vi "pop camera error.vi"(8 "error in (no error)":errorcluster, 11 "Channel in":refnum<class "Channel.lvclass">) -> (0 "error out":errorcluster, 2 "error":errorcluster, 3 "Channel out":refnum<class "Channel.lvclass">)   [LabVIEW 2018, in "Channel.lvclass"]
uses:
  Channel.lvclass
  Channel.lvclass/Channel.ctl
  Simulated_CCD_Camera/Simulated Camera.lvclass/Simulated Camera.ctl
  Simulated_CCD_Camera/Simulated Camera.lvclass
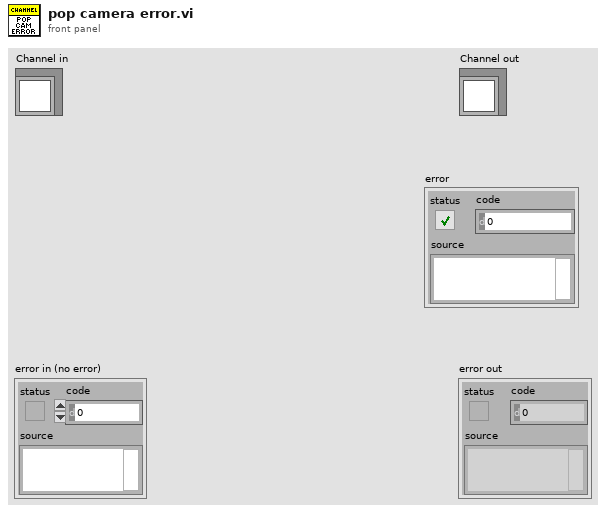
[diagram p1: front panel]
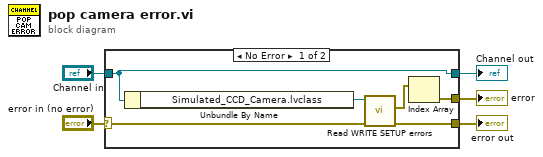
[diagram p0: block diagram]
diagram:
  n1 = case shown="No Error" "error in (no error)" {
    selector: "error in (no error)" -> [w9 w13]
    tunnel: [w8 w13] -> w4
    tunnel: [w11 w12] -> w2
    tunnel: "Channel in" -> [w11 w12]
    tunnel: [w6 _] -> w1
    frame No Error {
      n2 = Unbundle By Name(w11) -> ("Simulated_CCD_Camera.lvclass"=w10:refnum<class "Simulated Camera.lvclass">)
      n3 = call "Read WRITE SETUP errors.vi"("error in (no error)"=w9, "Simulated_CCD_Camera in"=w10) -> ("error out"=w8:errorcluster, "WRITE SETUP errors"=w7:errorcluster[])  [unwired: 7 in, 1 out]
      n4 = Index Array(array=w7) -> (element=w6:errorcluster)  [unwired: 1 in]
    }
    frame Error {
    }
  }
  "error out" <- w4
  "Channel out" <- w2
  "error" <- w1
